vi "Connect_SignatureIn_Signal.vi"(4 "Relay Signal Signature":string, 6 "Relay Object":refnum<class "LQObject.lvclass">, 8 "Error In":errorcluster, 10 "Source Signal Signature":string, 11 "Sender In":refnum<class "LQObject.lvclass">) -> (0 "Error Out":errorcluster, 3 "Sender Out":refnum<class "LQObject.lvclass">)   [LabVIEW 2013, in "Template.lvlib" / "LQCoreEngine.lvclass"]
uses:
  LQCoreEngine.lvclass
  LQObject/LQObject.lvclass
  LQIdentity/LQIdentity.lvclass/LQIdentity.ctl
  _Private/Signals and Slots/Relay Signal (Void).vi
  _Private/Signals and Slots/Relay Signal (Bool).vi
  _Private/Signals and Slots/Relay Signal (I32).vi
  _Private/Signals and Slots/Relay Signal (DBL).vi
  _Private/Signals and Slots/Relay Signal (String).vi
  LQIdentity/LQIdentity.lvclass
  Template.lvlib
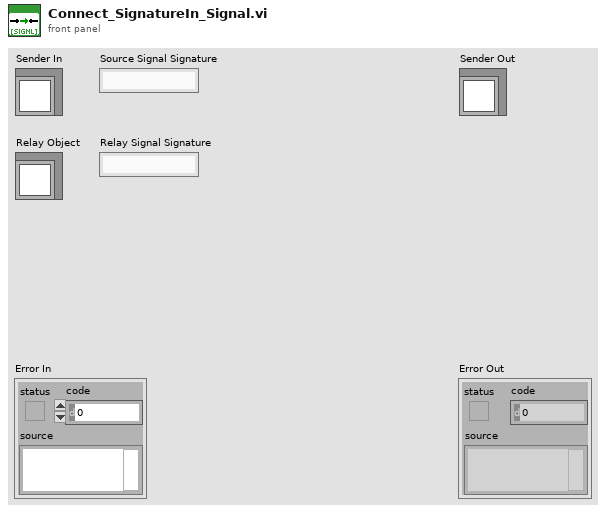
[diagram p1: front panel]
types:
  T1 = cluster{"Relay Object Refnum":u64, "Signal Index":i32}
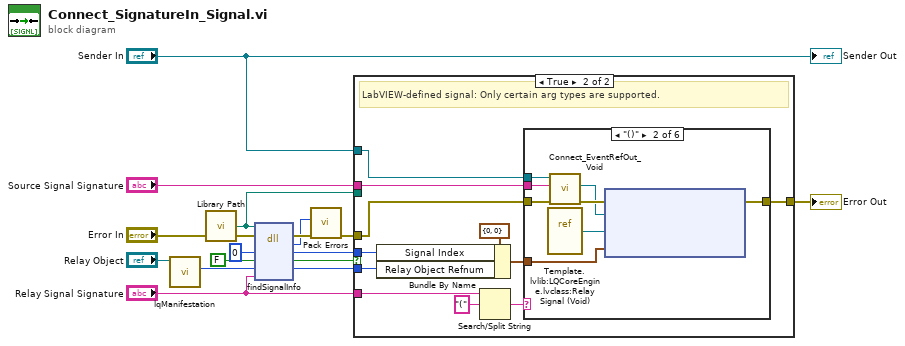
[diagram p0: block diagram]
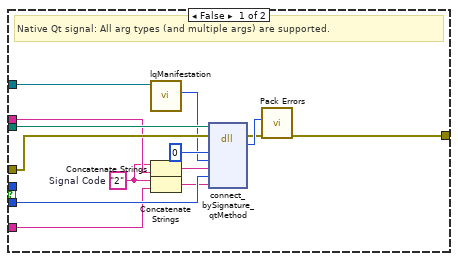
[diagram p2: hidden frame]
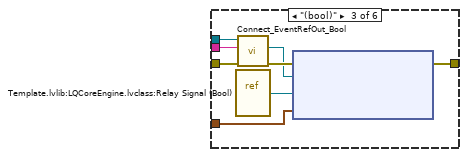
[diagram p4: hidden frame]
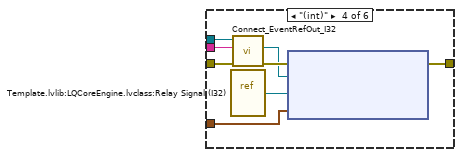
[diagram p5: hidden frame]
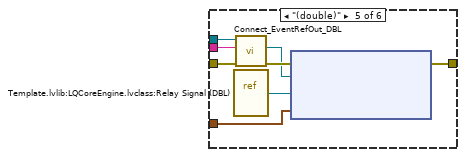
[diagram p6: hidden frame]
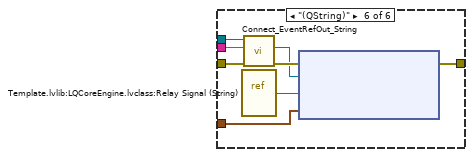
[diagram p7: hidden frame]
diagram:
  n1 = call "lqManifestation.vi"("LQIdentity in"="Relay Object") -> ("Manifestation"=w14:u64)  [unwired: 9 in, 1 out]
  n2 = call "Library Path.vi"() -> ("Library Path"=w7:path)
  n3 = dll-call lib="?" fn="findSignalInfo"(path in=w7, error in="Error In", "_retVal_signalIndex"=0, "_retVal_isDynamic"=FALSE, "_instance"=w14, "normalizedSignal"="Relay Signal Signature") -> (error out=w12:errorcluster, "errorCode"=w11:i32, "_retVal_signalIndex"=w9:i32, "_retVal_isDynamic"=w10:bool, "_instance"=w8:u64)  [unwired: 2 in, 1 out]
  n4 = call "Pack Errors.vi"("Error In"=w12, "Error Code"=w11) -> ("Error Out"=w6:errorcluster)  [unwired: 9 in]
  n5 = case shown="True" w10 {
    tunnel: w9 -> [_ w33]
    tunnel: w8 -> [w26 w32]
    tunnel: w7 -> [w27 _]
    tunnel: "Relay Signal Signature" -> [w25 w38]
    tunnel: w6 -> [w23 w37]
    tunnel: [w22 w35] -> w4
    tunnel: "Source Signal Signature" -> [w21 w36]
    tunnel: "Sender In" -> [w18 w39]
    frame False {
      w20 = "2"  # Signal Code
      # "Native Qt signal: All arg types (and multiple args) are supported."
      n6 = call "lqManifestation.vi"("LQIdentity in"=w18) -> ("Manifestation"=w17:u64)  [unwired: 9 in, 1 out]
      n7 = Concatenate Strings(w20, w21) -> (w19:string)
      n8 = Concatenate Strings(w20, w25) -> (w24:string)
      n9 = dll-call lib="?" fn="connect_bySignature_qtMethod"(path in=w27, error in=w23, "_retVal"=u64 0, "sender"=w17, "encodedSignal"=w19, "receiver"=w26, "encodedMethod"=w24) -> (error out=w29:errorcluster, "errorCode"=w30:i32)  [unwired: 6 in, 1 out]
      n10 = call "Pack Errors.vi"("Error In"=w29, "Error Code"=w30) -> ("Error Out"=w22:errorcluster)  [unwired: 9 in]
    }
    frame True {
      # "LabVIEW-defined signal: Only certain arg types are supported."
      n11 = Bundle By Name(cluster=T1 {"Relay Object Refnum"=0, "Signal Index"=0} ("User Parameter"), "Signal Index"=w33, "Relay Object Refnum"=w32) -> (w31:T1)
      n12 = Search/Split String(string=w38, search string/char (-)="(") -> (match + rest of string=w40:string)  [unwired: 1 in, 2 out]
      n13 = case shown="\"()\"" w40 {
        tunnel: w39 -> [_ w49 w57 w65 w73 w81]
        tunnel: w37 -> [w42 w48 w56 w64 w72 w80]
        tunnel: w36 -> [_ w47 w55 w63 w71 w79]
        tunnel: [w42 w44 w52 w60 w68 w76] -> w35
        tunnel: w31 -> [_ w43 w51 w59 w67 w75]
        frame Default {
          # "#TODO: Implement this check in C++\nLQApplication::finalizeBinding()"
          # "#ASSUMPTION: This case can't be\nreached because signals with unsupported\narg types can't be registered in the first\nplace. Thus, signals that use types not\nsupported by this innrt case structure will\nreturn FALSE for \"isDynamic\" anyway."
        }
        frame "()" {
          n14 = vi-ref "Template.lvlib:LQCoreEngine.lvclass:Relay Signal (Void).vi"() -> (w45:refnum<vi>)
          n15 = call "Connect_EventRefOut_Void.vi"("Error In"=w48, "Signal"=w47, "Sender In"=w49) -> ("Error Out"=w50:errorcluster, "Void Signal"=w46:refnum<user-event>)  [unwired: 6 in, 1 out]
          n16 = node(w50, w46, w45, w43) -> (w44:errorcluster)  [unwired: 1 in, 1 out]
        }
        frame "(bool)" {
          n17 = vi-ref "Template.lvlib:LQCoreEngine.lvclass:Relay Signal (Bool).vi"() -> (w53:refnum<vi>)
          n18 = call "Connect_EventRefOut_Bool.vi"("Error In"=w56, "Signal"=w55, "Sender In"=w57) -> ("Error Out"=w58:errorcluster, "Bool Signal"=w54:refnum<user-event>)  [unwired: 6 in, 1 out]
          n19 = node(w58, w54, w53, w51) -> (w52:errorcluster)  [unwired: 1 in, 1 out]
        }
        frame "(int)" {
          n20 = vi-ref "Template.lvlib:LQCoreEngine.lvclass:Relay Signal (I32).vi"() -> (w61:refnum<vi>)
          n21 = call "Connect_EventRefOut_I32.vi"("Error In"=w64, "Signal"=w63, "Sender In"=w65) -> ("Error Out"=w66:errorcluster, "I32 Signal"=w62:refnum<user-event>)  [unwired: 6 in, 1 out]
          n22 = node(w66, w62, w61, w59) -> (w60:errorcluster)  [unwired: 1 in, 1 out]
        }
        frame "(double)" {
          n23 = vi-ref "Template.lvlib:LQCoreEngine.lvclass:Relay Signal (DBL).vi"() -> (w69:refnum<vi>)
          n24 = call "Connect_EventRefOut_DBL.vi"("Error In"=w72, "Signal"=w71, "Sender In"=w73) -> ("Error Out"=w74:errorcluster, "DBL Signal"=w70:refnum<user-event>)  [unwired: 6 in, 1 out]
          n25 = node(w74, w70, w69, w67) -> (w68:errorcluster)  [unwired: 1 in, 1 out]
        }
        frame "(QString)" {
          n26 = vi-ref "Template.lvlib:LQCoreEngine.lvclass:Relay Signal (String).vi"() -> (w77:refnum<vi>)
          n27 = call "Connect_EventRefOut_String.vi"("Error In"=w80, "Signal"=w79, "Sender In"=w81) -> ("Error Out"=w82:errorcluster, "String Signal"=w78:refnum<user-event>)  [unwired: 6 in, 1 out]
          n28 = node(w82, w78, w77, w75) -> (w76:errorcluster)  [unwired: 1 in, 1 out]
        }
      }
    }
  }
  "Error Out" <- w4
  "Sender Out" <- "Sender In"
